vi "Brute Force Point Processing.  In Progress..vi"() -> ()   [LabVIEW 2016]
uses:
  Enums/Desired Points.ctl
  <vilib>/platform/TimedLoop/XDataNode/XDataNode.xnode
  <vilib>/Platform/TimedLoop/XDataNode/timing_clust.ctl
  <vilib>/Platform/TimedLoop/XDataNode/XDNodeRunTimeDep.lvlib
  <vilib>/Platform/TimedLoop/XDataNode/wakeup.ctl
  <vilib>/Platform/TimedLoop/XDataNode/nitl_modes.ctl
panel:
  in  "X pos Start":dbl
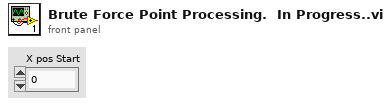
[diagram p1: front panel]
types:
  T1 = typedef "Desired Points.ctl" = enum16{"Hopper", "mid 1", "mid 2", "mid 3"}
  T2 = typedef "XDNodeRunTimeDep.lvlib/timing_clust.ctl" = cluster{"Expected End [f-1]":u64, "Actual End [f-1]":u64, "Finished Late? [f-1]":bool, "Expected End [i-1]":u64, "Actual End [i-1]":u64, "Finished Late? [i-1]":bool, "Expected Start [i]":u64, "Actual Start [i]":u64, "Expected Start [f]":u64, "Actual Start [f]":u64, "Source Name":string, "Structure Name":string, "Period":i64, "Deadline":i64, "Offset":i64, "Start":i64, "Priority":i32, "Timeout":i32, "Mode":T3, "Wakeup Reason":T4, "Error":errorcluster, "Source Type":string, "Secondary Source Type":string, "Global End Time":u64, "Global Start Time":u64, "Frame Duration":u64, "Iteration Duration":u64, "Assigned CPU":i32, "I/O Scan Engine Mode":u32}
  T3 = typedef "XDNodeRunTimeDep.lvlib/nitl_modes.ctl" = enum32{"No Change", "Process missed periods, maintain original phase", "Discard missed periods, maintain original phase", "Process missed periods, ignore original phase", "Discard missed periods, ignore original phase"}
  T4 = typedef "XDNodeRunTimeDep.lvlib/wakeup.ctl" = enum32{"Normal", "Aborted", "Asynchronous wakeup", "Timing source error", "Timed loop error", "Timeout"}
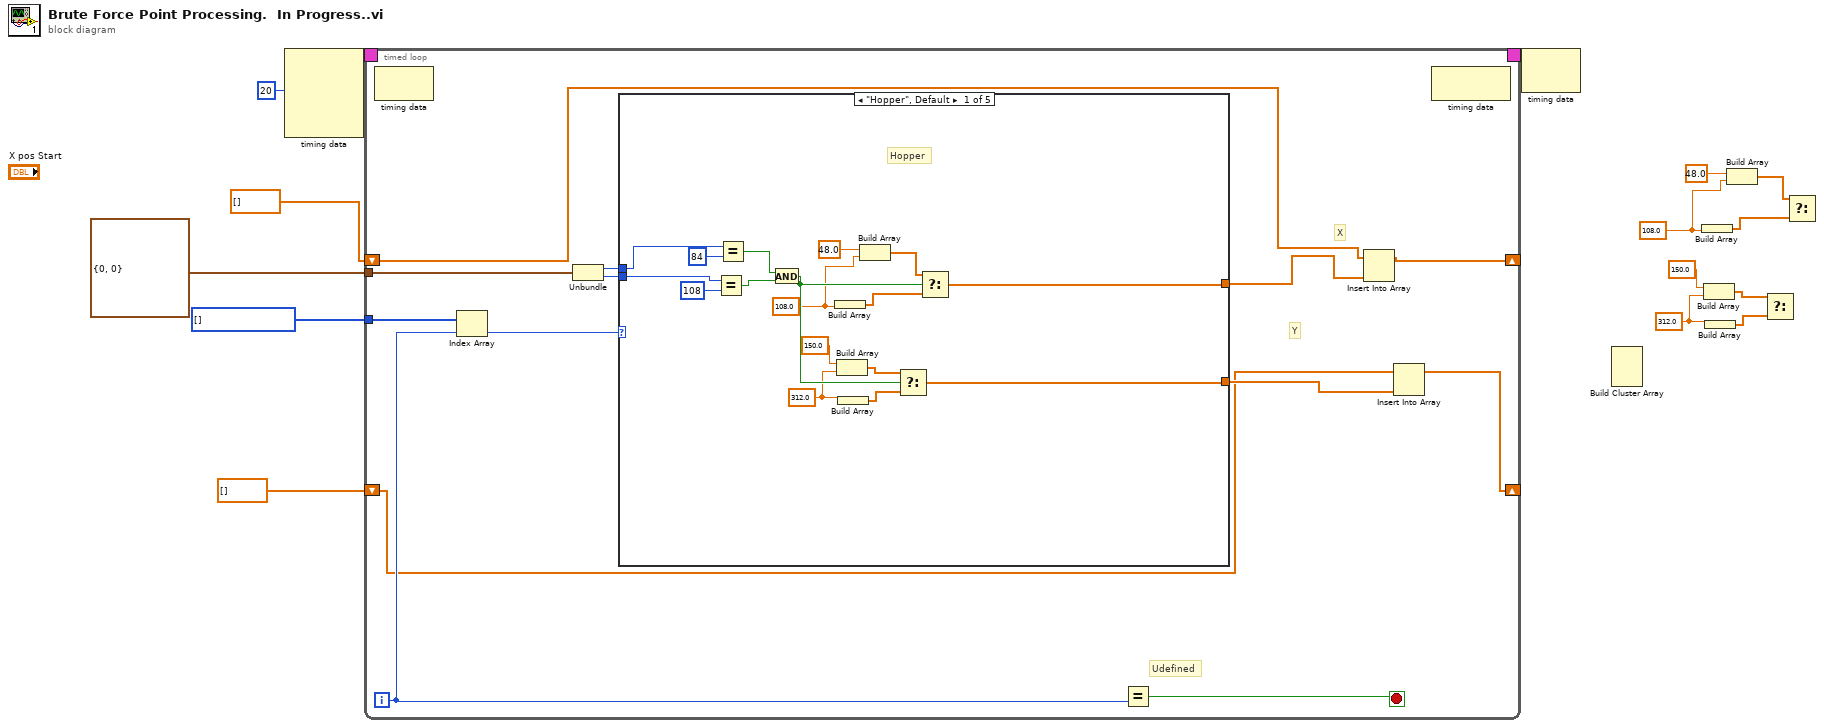
[diagram p0: block diagram]
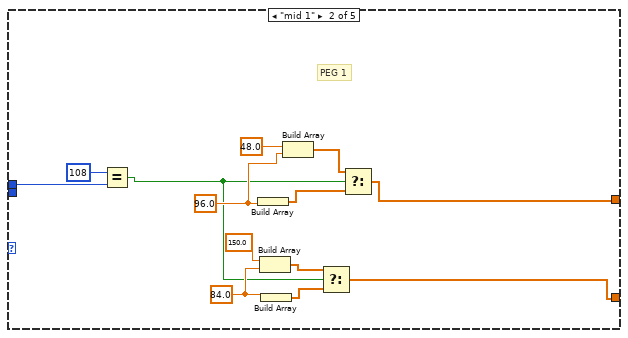
[diagram p2: hidden frame]
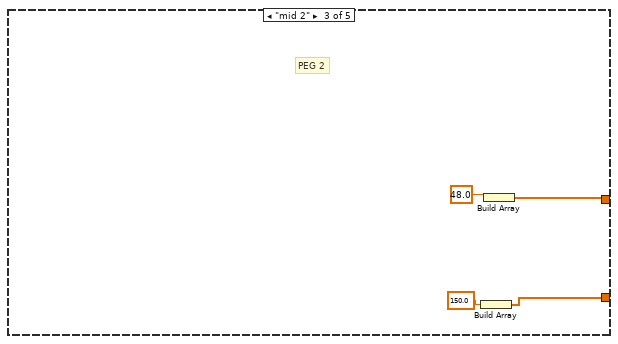
[diagram p3: hidden frame]
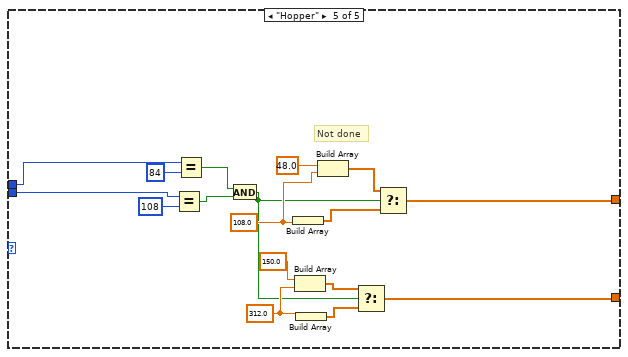
[diagram p5: hidden frame]
diagram:
  w3 = 312.0
  w6 = 108.0
  w15 = T1[] [] items=["Hopper", "mid 1", "mid 2", "mid 3"]
  n1 = node-c288(i64 20 ("Period")) -> (w13:T2)  [unwired: 3 in]
  n2 = timed-loop {
    tunnel: w15 -> [w28]
    tunnel: cluster{i32, i32} {0, 0} -> [w26]
    timing: w13 -> [_]
    timing-out: [_] -> w12
    shift-right: [w21] -> _
    shift-left: dbl[] [] -> [w19]
    shift-right: [w18] -> _
    shift-left: dbl[] [] -> [w16]
    i -> [w22]
    stop <- w23 stop-if-true
    # "Y"
    # "X"
    # "Udefined"
    n3 = node-c288() -> ()  [unwired: 1 in, 1 out]
    n4 = Index Array(array=w28, index=w22) -> (element=w27:T1)
    n5 = Unbundle(w26) -> (w25:i32, w24:i32)
    n6 = case shown="\"Hopper\", Default" w27 {
      tunnel: w25 -> [w47 w50 _ _ w68]
      tunnel: w24 -> [w44 _ _ _ w67]
      tunnel: [w41 w52 w63 _ w66] -> w20
      tunnel: [w39 w51 w64 _ w65] -> w17
      frame "Hopper", Default {
        w36 = 312.0
        w33 = 108.0
        # "Hopper"
        n7 = Equal?(x=w44, y=108) -> (x = y?=w42:bool)
        n8 = Equal?(x=w47, y=84) -> (x = y?=w43:bool)
        n9 = And(x=w43, y=w42) -> (x .and. y?=w40:bool)
        n10 = Build Array(w33) -> (w32:dbl[])
        n11 = Build Array(150.0, w36) -> (w37:dbl[])
        n12 = Build Array(w36) -> (w35:dbl[])
        n13 = Build Array(48.0, w33) -> (w31:dbl[])
        n14 = Select(t=w37, s=w40, f=w35) -> (s? t:f=w39:dbl[])
        n15 = Select(t=w31, s=w40, f=w32) -> (s? t:f=w41:dbl[])
      }
      frame "mid 1" {
        w58 = 84.0
        w55 = 96.0
        # "PEG 1"
        n16 = Equal?(x=108, y=w50) -> (x = y?=w48:bool)
        n17 = Build Array(w55) -> (w54:dbl[])
        n18 = Build Array(150.0, w58) -> (w59:dbl[])
        n19 = Build Array(w58) -> (w57:dbl[])
        n20 = Build Array(48.0, w55) -> (w53:dbl[])
        n21 = Select(t=w59, s=w48, f=w57) -> (s? t:f=w51:dbl[])
        n22 = Select(t=w53, s=w48, f=w54) -> (s? t:f=w52:dbl[])
      }
      frame "mid 2" {
        # "PEG 2"
        n23 = Build Array(150.0) -> (w64:dbl[])
        n24 = Build Array(48.0) -> (w63:dbl[])
      }
      frame "mid 3" {
      }
      frame "Hopper" {
        w76 = 312.0
        w79 = 108.0
        # "Not done"
        n25 = Equal?(x=w67, y=108) -> (x = y?=w72:bool)
        n26 = Equal?(x=w68, y=84) -> (x = y?=w71:bool)
        n27 = And(x=w71, y=w72) -> (x .and. y?=w73:bool)
        n28 = Build Array(w79) -> (w80:dbl[])
        n29 = Build Array(150.0, w76) -> (w75:dbl[])
        n30 = Build Array(w76) -> (w77:dbl[])
        n31 = Build Array(48.0, w79) -> (w81:dbl[])
        n32 = Select(t=w75, s=w73, f=w77) -> (s? t:f=w65:dbl[])
        n33 = Select(t=w81, s=w73, f=w80) -> (s? t:f=w66:dbl[])
      }
    }
    n34 = Equal?(y=w22) -> (x = y?=w23:bool)  [unwired: 1 in]
    n35 = Insert Into Array(array=w19, new element=w20) -> (w21:dbl[])  [unwired: 1 in]
    n36 = Insert Into Array(array=w16, new element=w17) -> (w18:dbl[])  [unwired: 1 in]
    n37 = node-c288() -> ()  [unwired: 1 in, 1 out]
  }
  n38 = node-c288(w12) -> ()  [unwired: 1 out]
  n39 = Build Cluster Array() -> ()  [unwired: 5 in, 1 out]
  n40 = Build Array(w6) -> (w7:dbl[])
  n41 = Build Array(150.0, w3) -> (w2:dbl[])
  n42 = Build Array(w3) -> (w4:dbl[])
  n43 = Build Array(48.0, w6) -> (w8:dbl[])
  n44 = Select(t=w2, f=w4) -> ()  [unwired: 1 in, 1 out]
  n45 = Select(t=w8, f=w7) -> ()  [unwired: 1 in, 1 out]
